vi "ReadNumbersWithCommas.vi"(8 "error in":errorcluster, 11 "file (use dialog)":path) -> (0 "error out":errorcluster, 1 "comma?":bool, 2 "text":string, 3 "fixed":string)   [LabVIEW 2022 SP3]
uses:
  Mic/Mic_Global.vi
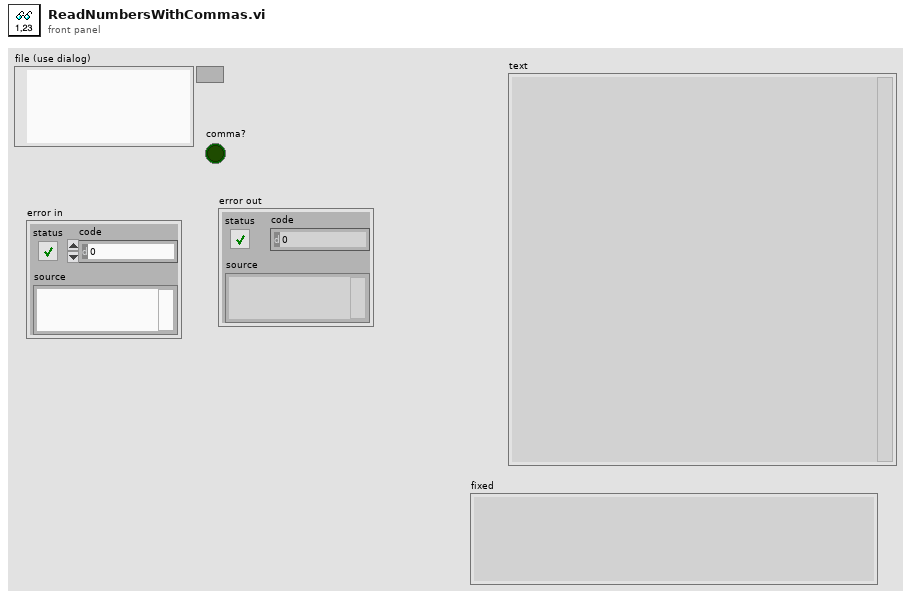
[diagram p1: front panel]
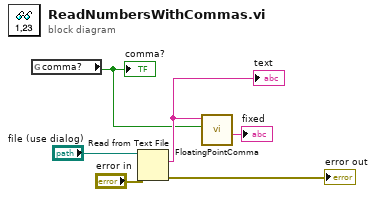
[diagram p0: block diagram]
diagram:
  n1 = global read "Mic_Global.vi" "comma?"() -> (w2:bool)
  "comma?" <- w2
  n2 = Read from Text File(file (use dialog)="file (use dialog)", error in="error in") -> (text=w3:string, error out=→"error out":errorcluster)  [unwired: 2 in, 2 out]
  "text" <- w3
  n3 = call "FloatingPointComma.vi"("Comma?"=w2, "String In"=w3) -> ("fixed"=→"fixed":string)  [unwired: 8 in, 1 out]
